vi "Add.vi"(8 "error in (no error)":errorcluster, 10 "Module ID":i32=-1, 11 "CloneRegRef":refnum<data-value>) -> (0 "error out":errorcluster, 2 "First?":bool, 3 "CloneRegRef":refnum<data-value>)   [LabVIEW 2018, in "ModuleAdmin.lvlib" / "CloneRegistration.lvclass"]
uses:
  CloneRegistration.lvclass
  CloneRegistration.lvclass/CloneRegistration.ctl
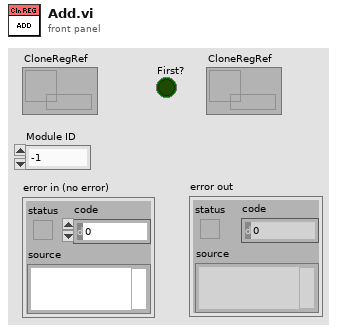
[diagram p1: front panel]
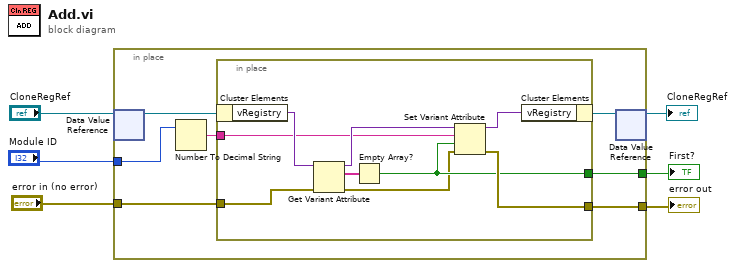
[diagram p0: block diagram]
diagram:
  n1 = in-place {
    in-place-border: "Module ID" -> [w11]
    in-place-border: "error in (no error)" -> [w10]
    in-place-border: [w8] -> w2
    in-place-border: [w7] -> w1
    n2 = in-place-dvr #1("CloneRegRef") -> (w12:refnum<class "CloneRegistration.lvclass">)  [unwired: 1 out]
    n3 = Number To Decimal String(number=w11) -> (decimal integer string=w13:string)  [unwired: 1 in]
    n4 = in-place {
      in-place-border: w13 -> [w19]
      in-place-border: w10 -> [w17]
      in-place-border: [w16] -> w7
      in-place-border: [w15] -> w8
      n5 = in-place-cluster #2(w12) -> ("vRegistry"=w21:variant)
      n6 = Get Variant Attribute(Variant=w21, error in=w17) -> (duplicate Variant=w20:variant, names=w22:string[], error out=w14:errorcluster)  [unwired: 2 in, 1 out]
      n7 = Empty Array?(array=w22) -> (empty?=w15:bool)
      n8 = Set Variant Attribute(Variant=w20, name=w19, value=w15, error in=w14) -> (Variant out=w18:variant, error out=w16:errorcluster)  [unwired: 1 out]
      n9 = in-place-cluster #2("vRegistry"=w18) -> (w9:refnum<class "CloneRegistration.lvclass">)
    }
    n10 = in-place-dvr #1(w9) -> (→"CloneRegRef":refnum<data-value>)  [unwired: 1 out]
  }
  "error out" <- w1
  "First?" <- w2
